vi "FPGA Acquire.vi"(0 "Logging queue in":T6, 1 "Max allowed trial length (sec)":dbl=15.0 format="%#_13g", 5 "Logging queue element":T3={"Imaging Protocol"=enum."Live Imaging", "Number of Trials"=0, "Frame Size"=512, "# Averaged frames"=0, "Dwell time (us)"=0.0, "Index of Z-plane"=0, "Timelapse?"=FALSE, "Logging process is active"=FALSE, "Speed logging enabled"=FALSE, "tdms file ref"=refnum, "path"=path "", "Trial Number"=0, "Expected # points acquired"=FALSE, "Manually stopped"=FALSE, "Last trial"=FALSE, "Ch0 data"=[], "Ch1 data"=[], "Ref Data"=[], "Ref Frame Time"=[], "Image Time"=[], "Continuous Time"=[], "Ref X Length"=0, "Ref Y Length"=0, "# Ref Averaged frames"=0, "Ref Dwell time (us)"=0.0, "Points acquired"={"Ch0 last trial"=0, "Ch1 last trial"=0, "All trials"=0}, "HW Timings File"=refnum} {"Ref Dwell time (us)" format="%#.6g"; "Frame Size" items=["100X100"=100, "128X128"=128, "200X200"=200, "256X256"=256, "512X512"=512, "1024x1024"=1024, "2048x2048"=2048]; "Dwell time (us)" format="%#.6g"}, 7 "FPGA Ref":T2, 9 "Target number of points":u64, 11 "error in (no error)":errorcluster, 12 "Total number of Ref points":u32, 13 "Imaging Protocol":T1) -> (4 "Logging queue out":T6, 6 "Logging queue element":T3={"Imaging Protocol"=enum."Live Imaging", "Number of Trials"=0, "Frame Size"=512, "# Averaged frames"=0, "Dwell time (us)"=0.0, "Index of Z-plane"=0, "Timelapse?"=FALSE, "Logging process is active"=FALSE, "Speed logging enabled"=FALSE, "tdms file ref"=refnum, "path"=path "", "Trial Number"=0, "Expected # points acquired"=FALSE, "Manually stopped"=FALSE, "Last trial"=FALSE, "Ch0 data"=[], "Ch1 data"=[], "Ref Data"=[], "Ref Frame Time"=[], "Image Time"=[], "Continuous Time"=[], "Ref X Length"=0, "Ref Y Length"=0, "# Ref Averaged frames"=0, "Ref Dwell time (us)"=0.0, "Points acquired"={"Ch0 last trial"=0, "Ch1 last trial"=0, "All trials"=0}, "HW Timings File"=refnum} {"Ref Dwell time (us)" format="%#.6g"; "Frame Size" items=["100X100"=100, "128X128"=128, "200X200"=200, "256X256"=256, "512X512"=512, "1024x1024"=1024, "2048x2048"=2048]; "Dwell time (us)" format="%#.6g"}, 8 "Elements Remaining":u32, 10 "VI exec time":u32, 15 "error out":errorcluster)   [LabVIEW 2020]
uses:
  Typedefs/Logging queue element.ctl
  Typedefs/Imaging Protocols enum.ctl
  Typedefs/Frame Size.ctl
  Typedefs/Acquired points count.ctl
  Typedefs/Data queue ref.ctl
  RIG-SPECIFIC FILES/FPGA Refs/FPGA Ref.ctl
panel:
  out "Array":u32[](array[numeric])
  out "Ref Elements Remaining":u32
  out "# elements in queue":i32
  out "VI exec interval":u32
  out "Execution rate (Hz) 3":i32 format="Execution Rate: %.0f Hz"
  out "Execution rate (Hz)":i32 format="Execution Rate: %.0f Hz"
  out "Trial completed or \nImaging stopped":bool
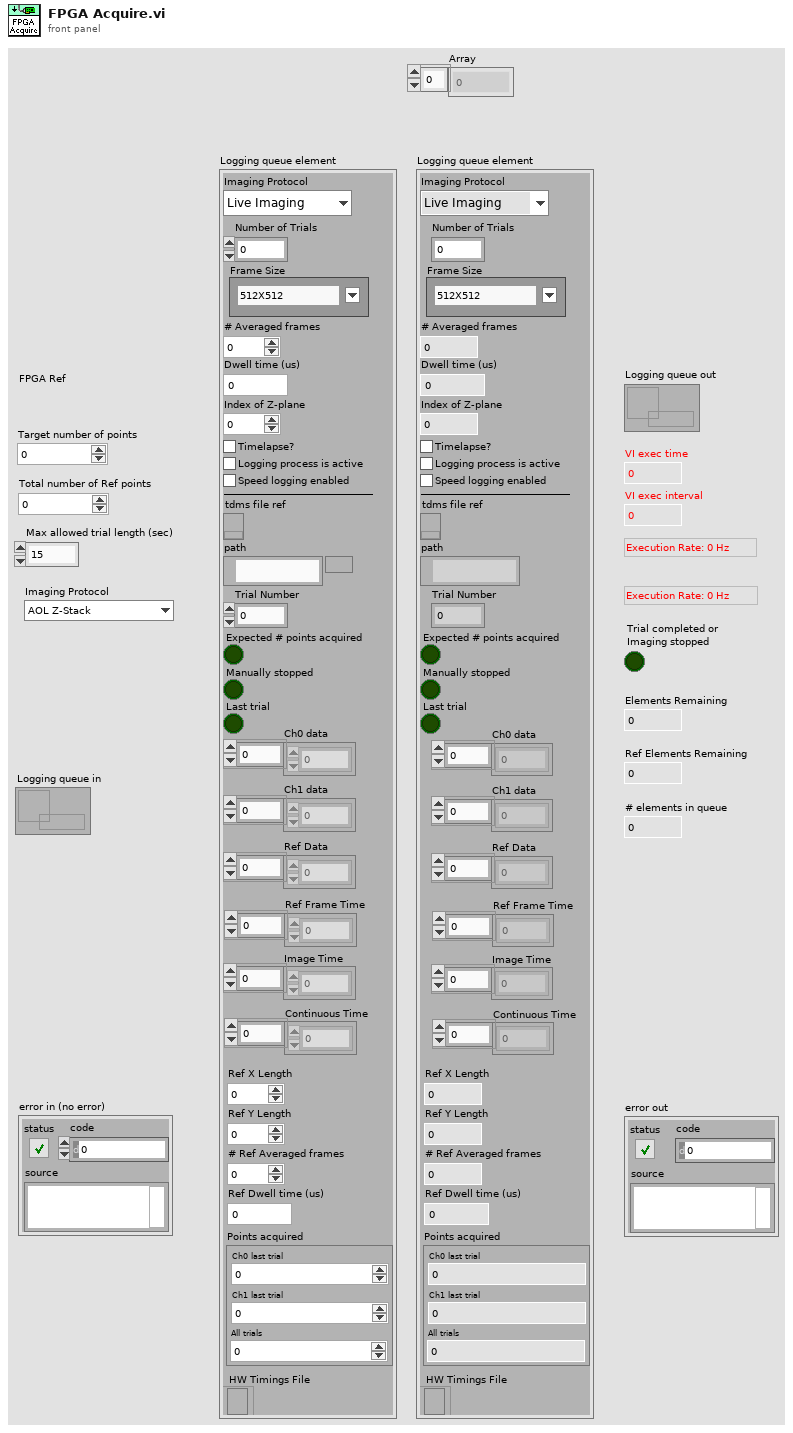
[diagram p1: front panel]
types:
  T1 = typedef "Imaging Protocols enum.ctl" = enum16{"AOL Z-Stack", "Motor Z Stack", "Functional Acquisition", "Single Plane Acquisition", "Volume Acquisition", "Live Imaging", "Live Plane Imaging", "Live Volume Imaging"}
  T2 = typedef "FPGA Ref.ctl" = refnum<k20>
  T3 = typedef "Logging queue element.ctl" = cluster{"Imaging Protocol":T1, "Number of Trials":u16, "Frame Size":T4, "# Averaged frames":u16, "Dwell time (us)":dbl, "Index of Z-plane":i32, "Timelapse?":bool, "Logging process is active":bool, "Speed logging enabled":bool, "tdms file ref":refnum<k34>, "path":path, "Trial Number":i32, "Expected # points acquired":bool, "Manually stopped":bool, "Last trial":bool, "Ch0 data":u32[], "Ch1 data":u32[], "Ref Data":u32[], "Ref Frame Time":u64[], "Image Time":u64[], "Continuous Time":u64[], "Ref X Length":u16, "Ref Y Length":u16, "# Ref Averaged frames":u16, "Ref Dwell time (us)":dbl, "Points acquired":T5, "HW Timings File":refnum<file>}
  T4 = typedef "Frame Size.ctl" = u16
  T5 = typedef "Acquired points count.ctl" = cluster{"Ch0 last trial":u64, "Ch1 last trial":u64, "All trials":u64}
  T6 = typedef "Data queue ref.ctl" = refnum<queue>
  T7 = typedef "FIFO elements available.ctl" = cluster{"Elements Available Ch0":u32, "Elements Available Ch1":u32, "Ref Elements Available":u32, "Ref Time Elements":u32, "Image Time Elements":u32, "Inter trial elements":u32}
  T8 = typedef "Data arrays cluster.ctl" = cluster{"Ch0 data":u32[], "Ch1 data":u32[], "Ref data":u32[], "Ref time data":u64[], "Image time data":u64[], "Continuous time data":u64[]}
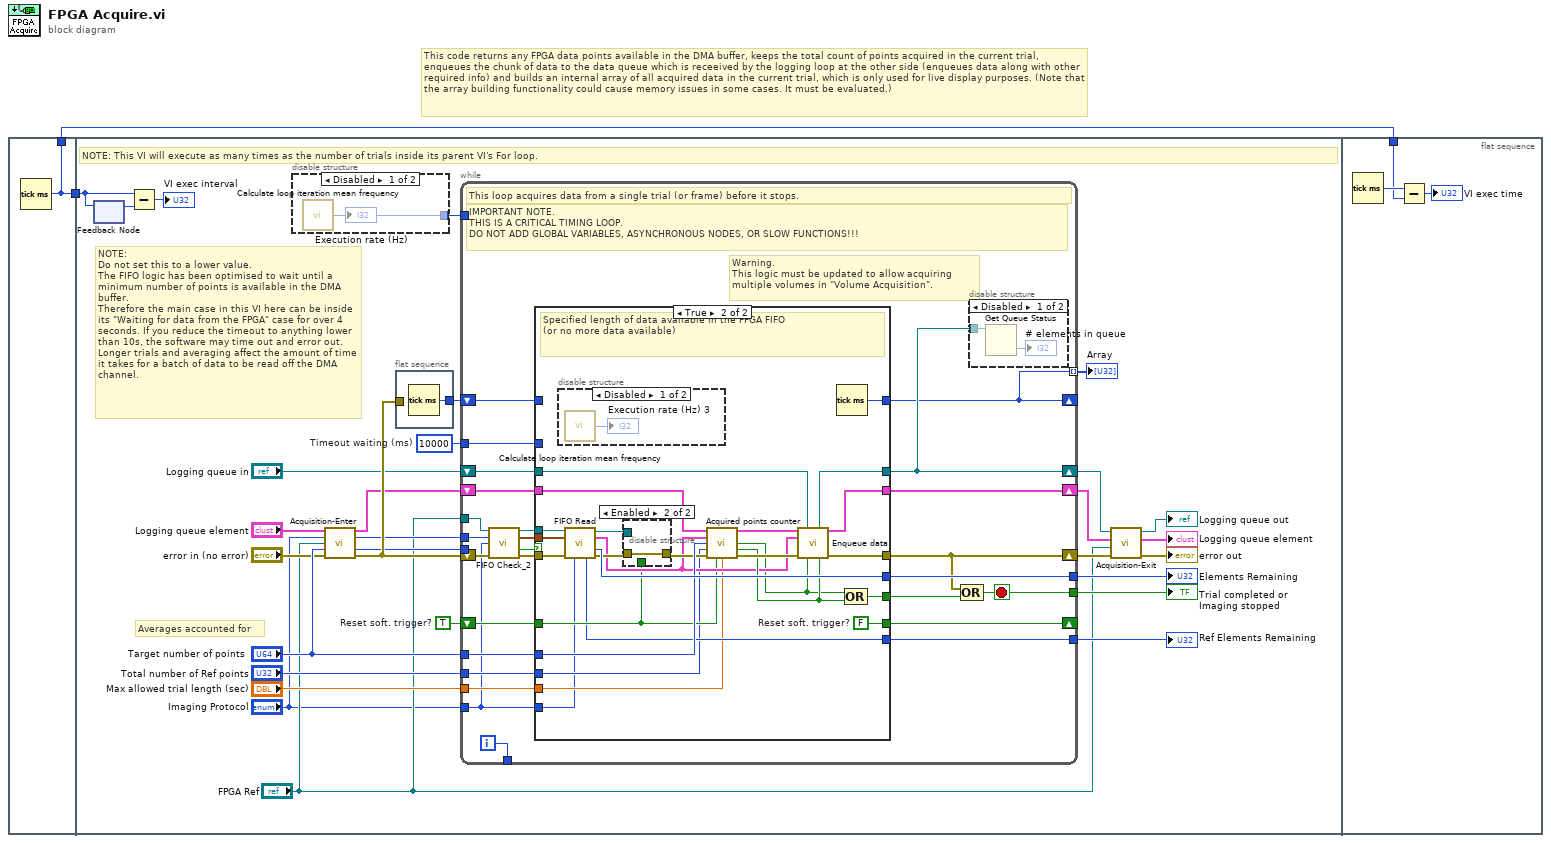
[diagram p0: block diagram]
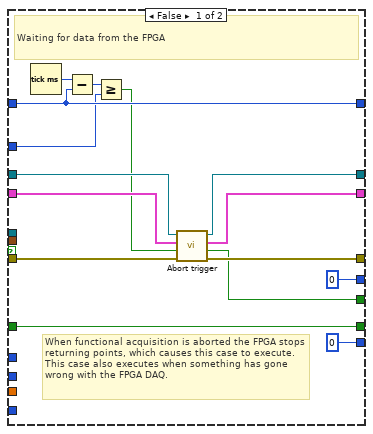
[diagram p4: hidden frame]
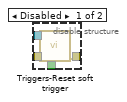
[diagram p5: hidden frame]
diagram:
  # "This code returns any FPGA data points available in the DMA buffer, keeps the total count of points acquired in the current trial, enqueues the chunk of data to the data queue which is receeived by the logging loop at the other side (enqueues data along with other required info) and builds an internal array of all acquired data in the current trial, which is only used for live display purposes. (Note that the array building functionality could cause memory issues in some cases. It must be evaluated.)"
  n1 = flat-sequence {
    tunnel: [w3] -> w1
    tunnel: [w3] -> w2
    tunnel: w2 -> [w22]
    tunnel: w1 -> [w110]
    frame #0 {
      n2 = Tick Count (ms)() -> (millisecond timer value=w3:u32)
    }
    frame #1 {
      w21 = TRUE  # Reset soft. trigger?
      w26 = u32 10000  # Timeout waiting (ms)
      # "NOTE:\nDo not set this to a lower value.\nThe FIFO logic has been optimised to wait until a minimum number of points is available in the DMA buffer.\nTherefore the main case in this VI here can be inside its \"Waiting for data from the FPGA\" case for over 4 seconds. If you reduce the timeout to anything lower than 10s, the software may time out and error out.\nLonger trials and averaging affect the amount of time it takes for a batch of data to be read off the DMA channel."
      # "Averages accounted for"
      # "NOTE: This VI will execute as many times as the number of trials inside its parent VI's For loop."
      n3 = feedback #1() -> (w24:u32)  [unwired: 1 in]
      n4 = feedback-in #1(w22) -> ()
      n5 = Subtract(x=w22, y=w24) -> (x-y=→"VI exec interval":u32)
      n6 = disable-structure shown="Disabled" {
        disable-tunnel: [w34 _] -> w25
        frame Disabled {
          n7 = call "Calculate loop iteration mean frequency.vi"() -> ("Refresh rate (Hz)"=w34:i32)  [unwired: 1 in]
          "Execution rate (Hz)" <- w34
        }
        frame Enabled {
        }
      }
      n8 = call "Acquisition-Enter.vi"("Logging queue element in"="Logging queue element", "Imaging Protocol"="Imaging Protocol", "FPGA Ref"="FPGA Ref", "Target number of points"="Target number of points", "error in (no error)"="error in (no error)") -> ("Logging queue element out"=w13:T3, "Read at least # points"=w20:u32, "Read at least # Ref points"=w19:u32, "error out"=w32:errorcluster)  [unwired: 7 in]
      n9 = flat-sequence {
        tunnel: [w33] -> w27
        tunnel: w32 -> [_]
        frame #0 {
          n10 = Tick Count (ms)() -> (millisecond timer value=w33:u32)
        }
      }
      n11 = while {
        tunnel: w19 -> [_]
        tunnel: [w42] -> w12
        tunnel: [w56] -> w30
        shift-right: [w49] -> w8
        shift-left: "Logging queue in" -> [w57]
        shift-right: [w40] -> w28
        shift-left: w32 -> [w60]
        tunnel: "FPGA Ref" -> [w54]
        tunnel: w25 -> [_]
        shift-right: [w35] -> _
        shift-left: w27 -> [w53]
        tunnel: w26 -> [w52]
        shift-right: [w50] -> _
        shift-left: w21 -> [w51]
        tunnel: "Target number of points" -> [w47]
        tunnel: w20 -> [w46]
        tunnel: [w45] -> w18
        tunnel: "Total number of Ref points" -> [w44]
        tunnel: "Max allowed trial length (sec)" -> [w43]
        shift-right: [w39] -> w9
        shift-left: w13 -> [w55]
        tunnel: [w38] -> _
        tunnel: "Imaging Protocol" -> [w36]
        tunnel: [w35] -> w4 mode=indexing
        i -> [w38]
        stop <- w42 stop-if-true
        # "IMPORTANT NOTE.\nTHIS IS A CRITICAL TIMING LOOP.\nDO NOT ADD GLOBAL VARIABLES, ASYNCHRONOUS NODES, OR SLOW FUNCTIONS!!!"
        # "Warning.\nThis logic must be updated to allow acquiring multiple volumes in \"Volume Acquisition\"."
        # "This loop acquires data from a single trial (or frame) before it stops."
        n12 = call "FIFO Check_2.vi"("FPGA Ref in"=w54, "Read at least # points"=w46, "Imaging Protocol"=w36, "error in (no error)"=w60) -> ("FPGA Ref out"=w59:T2, "Elements Available"=w37:T7, "Data available or data has just completed (read the FIFO)"=w48:bool, "error out"=w58:errorcluster)  [unwired: 7 in, 1 out]
        n13 = case shown="True" w48 {
          tunnel: w58 -> [w71 w98]
          tunnel: w59 -> [_ w100]
          tunnel: [w63 w93] -> w41
          tunnel: w47 -> [_ w95]
          tunnel: w55 -> [w65 w85]
          tunnel: w57 -> [w69 w83]
          tunnel: [w68 w82] -> w49
          tunnel: [w72 w94] -> w40
          tunnel: [u32 0 ("Elements Remaining") w103] -> w56
          tunnel: [w67 w80] -> w39
          tunnel: w53 -> [w74 _]
          tunnel: [w74 w101] -> w35
          tunnel: w52 -> [w73 _]
          tunnel: w51 -> [w70 w89]
          tunnel: [w70 w99] -> w50
          tunnel: [u32 0 ("Ref Elements Remaining") w88] -> w45
          tunnel: w44 -> [_ w87]
          tunnel: w43 -> [_ w86]
          tunnel: w37 -> [_ w79]
          tunnel: w36 -> [_ w78]
          frame False {
            # "When functional acquisition is aborted the FPGA stops returning points, which causes this case to execute. This case also executes when something has gone wrong with the FPGA DAQ."
            # "Waiting for data from the FPGA"
            n14 = Tick Count (ms)() -> (millisecond timer value=w75:u32)
            n15 = Subtract(x=w75, y=w74) -> (x-y=w76:u32)
            n16 = Greater Or Equal?(x=w76, y=w73) -> (x >= y?=w64:bool)
            n17 = call "Abort trigger.vi"("error in (no error)"=w71, "Timed out waiting on data"=w64, "Logging queue element in"=w65, "Logging queue in"=w69) -> ("error out"=w72:errorcluster, "Stop the acquisition module"=w63:bool, "Logging queue metadata shift out"=w67:T3, "Logging queue out"=w68:T6)  [unwired: 4 in]
          }
          frame True {
            w99 = FALSE  # Reset soft. trigger?
            # "Specified length of data available in the FPGA FIFO\n(or no more data available)"
            n18 = disable-structure shown="Disabled" {
              frame Disabled {
                n19 = call "Calculate loop iteration mean frequency.vi"() -> ("Refresh rate (Hz)"=→"Execution rate (Hz) 3":i32)  [unwired: 1 in]
              }
              frame Enabled {
              }
            }
            n20 = call "FIFO Read.vi"("FPGA Ref"=w100, "Elements Available"=w79, "error in"=w98, "Imaging Protocol"=w78) -> ("FPGA VI Reference Out"=w96:T2, "Data arrays cluster"=w90:T8, "Elements Remaining (Ch0)"=w103:u32, "Image Time Elements Remaining"=w88:u32, "error out"=w97:errorcluster)  [unwired: 7 in]
            n21 = disable-structure shown="Enabled" {
              disable-tunnel: w97 -> [w107 w108]
              disable-tunnel: w96 -> [w106 _]
              disable-tunnel: [w105 w108] -> w91
              disable-tunnel: w89 -> [w104 _]
              frame Disabled {
                n22 = call "Triggers-Reset soft trigger.vi"("Reset soft. trigger"=w104, "error in (no error)"=w107, "FPGA Ref"=w106) -> ("error out"=w105:errorcluster)  [unwired: 8 in]
              }
              frame Enabled {
              }
            }
            n23 = call "Acquired points counter.vi"("Logging queue element"=w85, "Raw Data Array"=w90, "Number of samples to be acquired (points in frame x Ch. x Av.)"=w95, "Number of Ref samples to be acquired"=w87, "error in"=w91, "Initial reset"=w89, "Max allowed trial length (sec)"=w86) -> ("Logging queue element"=w81:T3, "Expected number of funct.acq points acquired on both channels"=w84:bool, "Live imaging stopped"=w92:bool, "error out"=w102:errorcluster)  [unwired: 5 in]
            n24 = call "Enqueue data.vi"("Logging queue metadata shift in"=w81, "Logging queue in"=w83, "Chunk of data"=w90, "Error in"=w102, "Expected # points acquired"=w84, "Manually stopped"=w92) -> ("Logging queue out"=w82:T6, "Logging queue metadata shift out"=w80:T3, "error out"=w94:errorcluster)  [unwired: 7 in]
            n25 = Tick Count (ms)() -> (millisecond timer value=w101:u32)
            n26 = Compound Arithmetic op=OR(w84, w92) -> (w93:bool)
          }
        }
        n27 = Compound Arithmetic op=OR(w40, w41) -> (w42:bool)
        n28 = disable-structure shown="Disabled" {
          disable-tunnel: w49 -> [w62 _]
          frame Disabled {
            n29 = Get Queue Status(queue=w62) -> (# elements in queue=→"# elements in queue":i32)  [unwired: 2 in, 7 out]
          }
          frame Enabled {
          }
        }
      }
      "Elements Remaining" <- w30
      "Trial completed or \nImaging stopped" <- w12
      "Ref Elements Remaining" <- w18
      "Array" <- w4
      n30 = call "Acquisition-Exit.vi"("error in (no error)"=w28, "FPGA Ref"="FPGA Ref", "Logging queue element in"=w9, "Logging queue in"=w8) -> ("error out"=→"error out":errorcluster, "Logging queue element"=→"Logging queue element":T3, "Logging queue out"=→"Logging queue out":T6)  [unwired: 5 in]
    }
    frame #2 {
      n31 = Tick Count (ms)() -> (millisecond timer value=w111:u32)
      n32 = Subtract(x=w111, y=w110) -> (x-y=→"VI exec time":u32)
    }
  }
